vi "Browse to item in Windows Explorer.vi"(8 "error in (no error)":errorcluster, 11 "File":path) -> (0 "error out":errorcluster)   [LabVIEW 2011, in "COSYLib.lvlib"]
doc: "Opens Window Explorer in the location of the specified file, selecting the file."
uses:
  COSYLib.lvlib
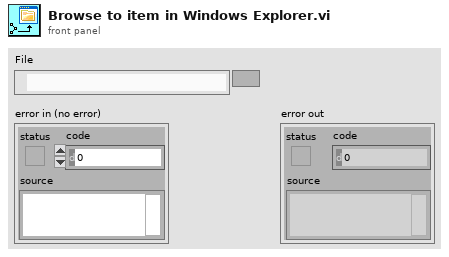
[diagram p1: front panel]
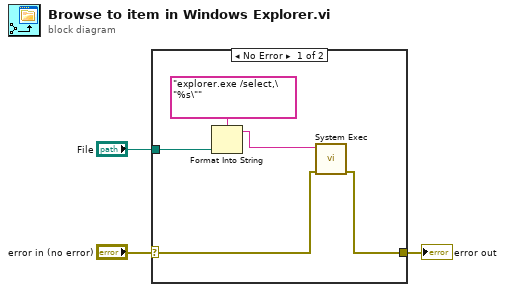
[diagram p0: block diagram]
diagram:
  n1 = case shown="No Error" "error in (no error)" {
    selector: "error in (no error)" -> [w5 w9]
    tunnel: [w4 w9] -> w2
    tunnel: "File" -> [w8 _]
    frame No Error {
      n2 = Format Into String(format string="explorer.exe /select,\"%s\"", w8) -> (resulting string=w7:string)  [unwired: 2 in, 1 out]
      n3 = call <vilib>:"System Exec.vi"("error in (no error)"=w5, "command line"=w7) -> ("error out"=w4:errorcluster)  [unwired: 6 in, 3 out]
    }
    frame Error {
    }
  }
  "error out" <- w2
